vi "wave 1.vi"() -> ()   [LabVIEW 2011]
panel:
  out "Waveform Chart":dbl[](graph)
  out "Waveform Graph":dbl[](graph)
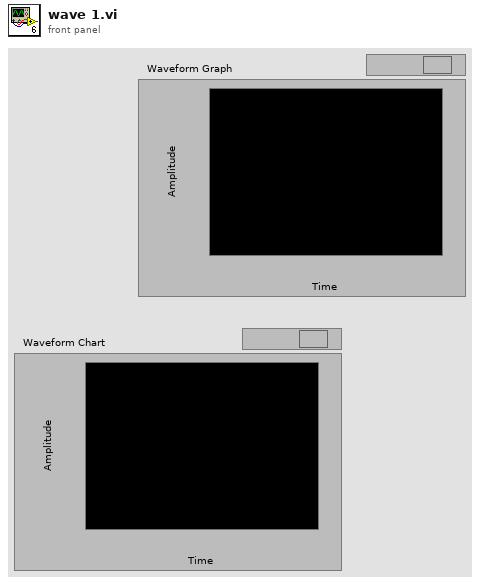
[diagram p1: front panel]
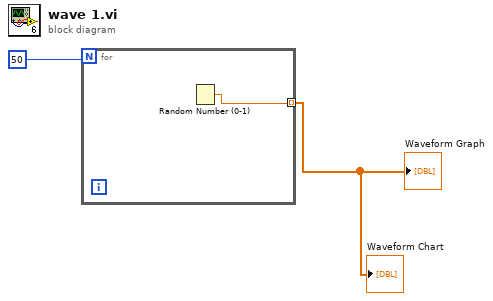
[diagram p0: block diagram]
diagram:
  n1 = for {
    N: 50 -> [_]
    tunnel: [w3] -> w1 mode=indexing
    n2 = Random Number (0-1)() -> (number: 0 to 1=w3:dbl)
  }
  "Waveform Graph" <- w1
  "Waveform Chart" <- w1
